vi "SQLite Get Calib.Parameters.vi"(8 "error in (no error)":errorcluster, 9 "VariableName":string, 10 "Order By":T1, 11 "Main":string="0") -> (0 "error out":errorcluster, 1 "Full Result":string[][](array[string]), 2 "Value":string, 3 "DBL Value":dbl, 4 "Results":string[](array[string]), 5 "Unit":string)   [LabVIEW 2017, in "SQLite.lvclass"]
doc: "get Calibration Parmeters.\n2015-11-05 10:00:32\n蒋松\njiangsong@outlook.com"
uses:
  SQLite.lvclass
  Order By.ctl
  SQLiteFileName.ctl
  TabelFullName.ctl
  <vilib>/Utility/error.llb/Trim Whitespace.vi
  <userlib>/LabSQL/LabSQL.lvlib
  <userlib>/sushu/sushu.lvlib
panel:
  in  "VI Ref":refnum<vi>
  in  "Alarm":bool=TRUE
  out "Boolean":bool
  in  "CMD":T2(ring)=enum."Read"
  out "Select SQL CMD":string
  # "Test-Force"
  # "ChannelItems"
  # "当是字符串格式的数字时，\n大于9后，排序会乱，\n1\n10\n2\n3\n...."
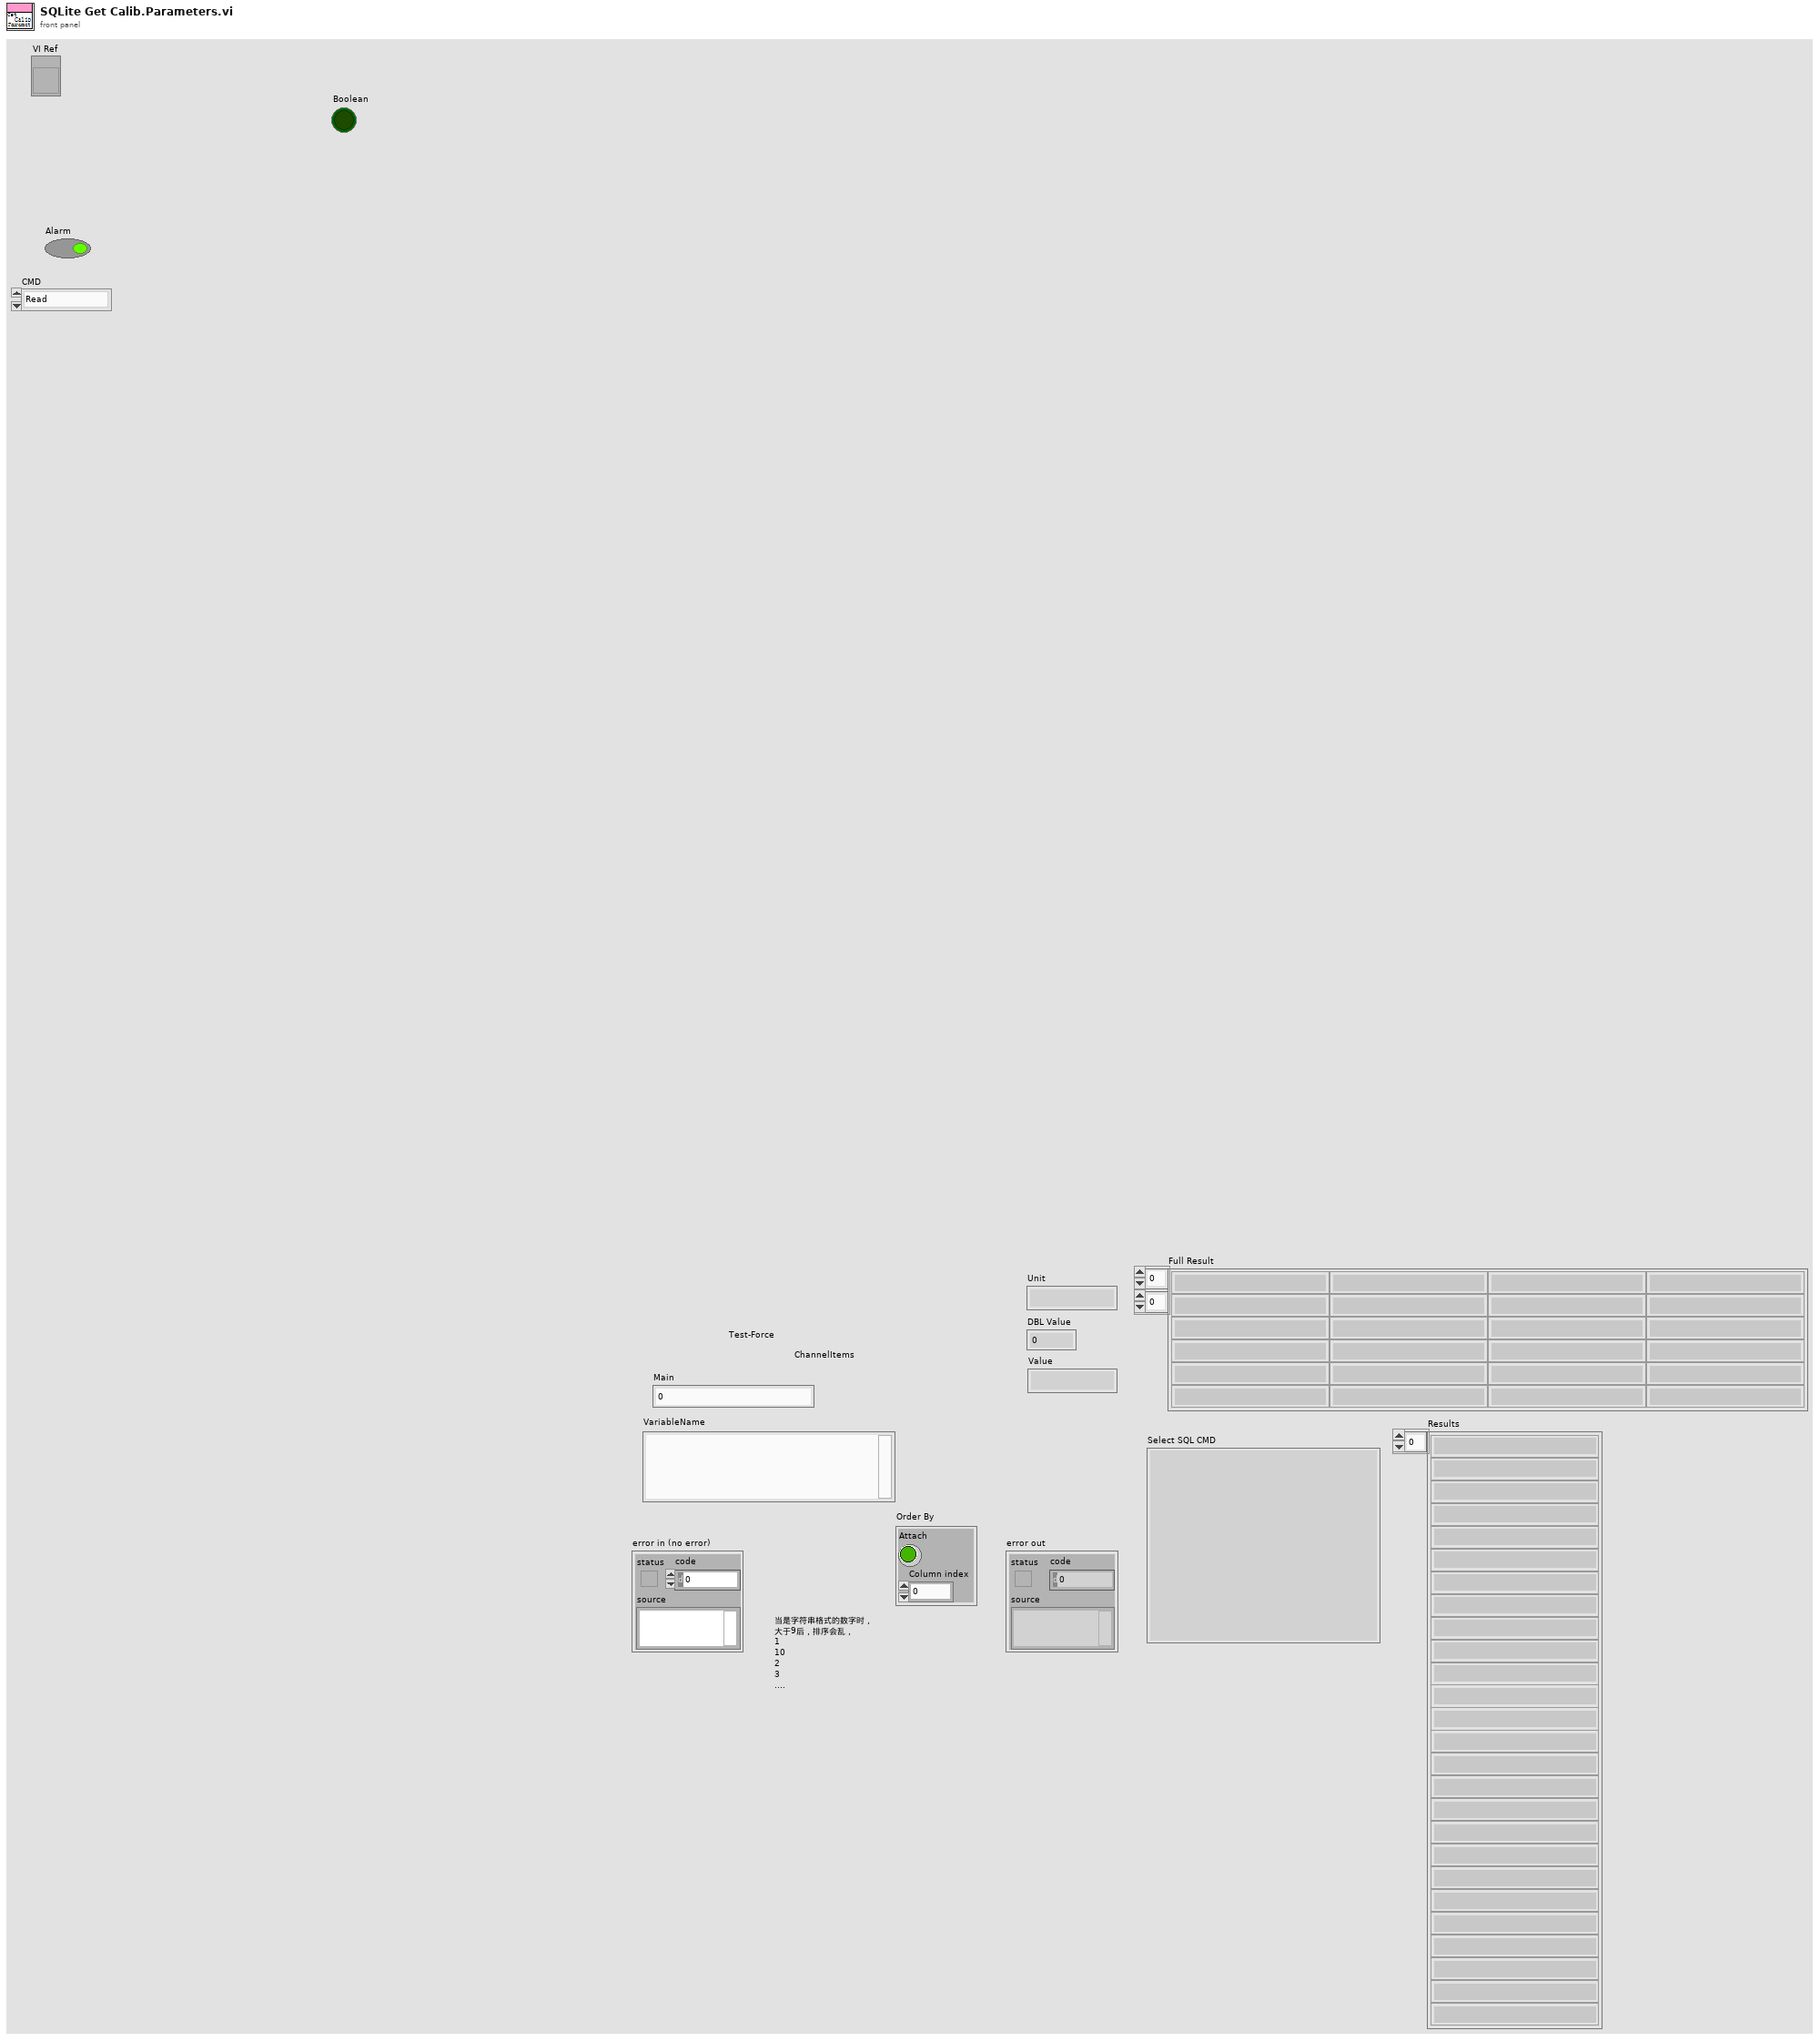
[diagram p1: front panel]
types:
  T1 = typedef "SQLite.lvclass/Order By.ctl" = cluster{"Attach":bool, "Column index":i32}
  T2 = enum16{"Initialize", "Read", "Write", "UnInitialize"}
  T3 = typedef "SQLite.lvclass/TabelFullName.ctl" = string
  T4 = typedef "SQLite.lvclass/SQLiteFileName.ctl" = string
  T5 = cluster{"Current VI Reference":refnum<vi>, "Close Panel on Exit?":bool}
  T6 = cluster{"Core":cluster{"Current VI Reference":refnum<vi>, "Close Panel on Exit?":bool}, "VI Name":string}
  T7 = enum16{"Other", "SQL2008", "SQLite", "Access", "MySQL"}
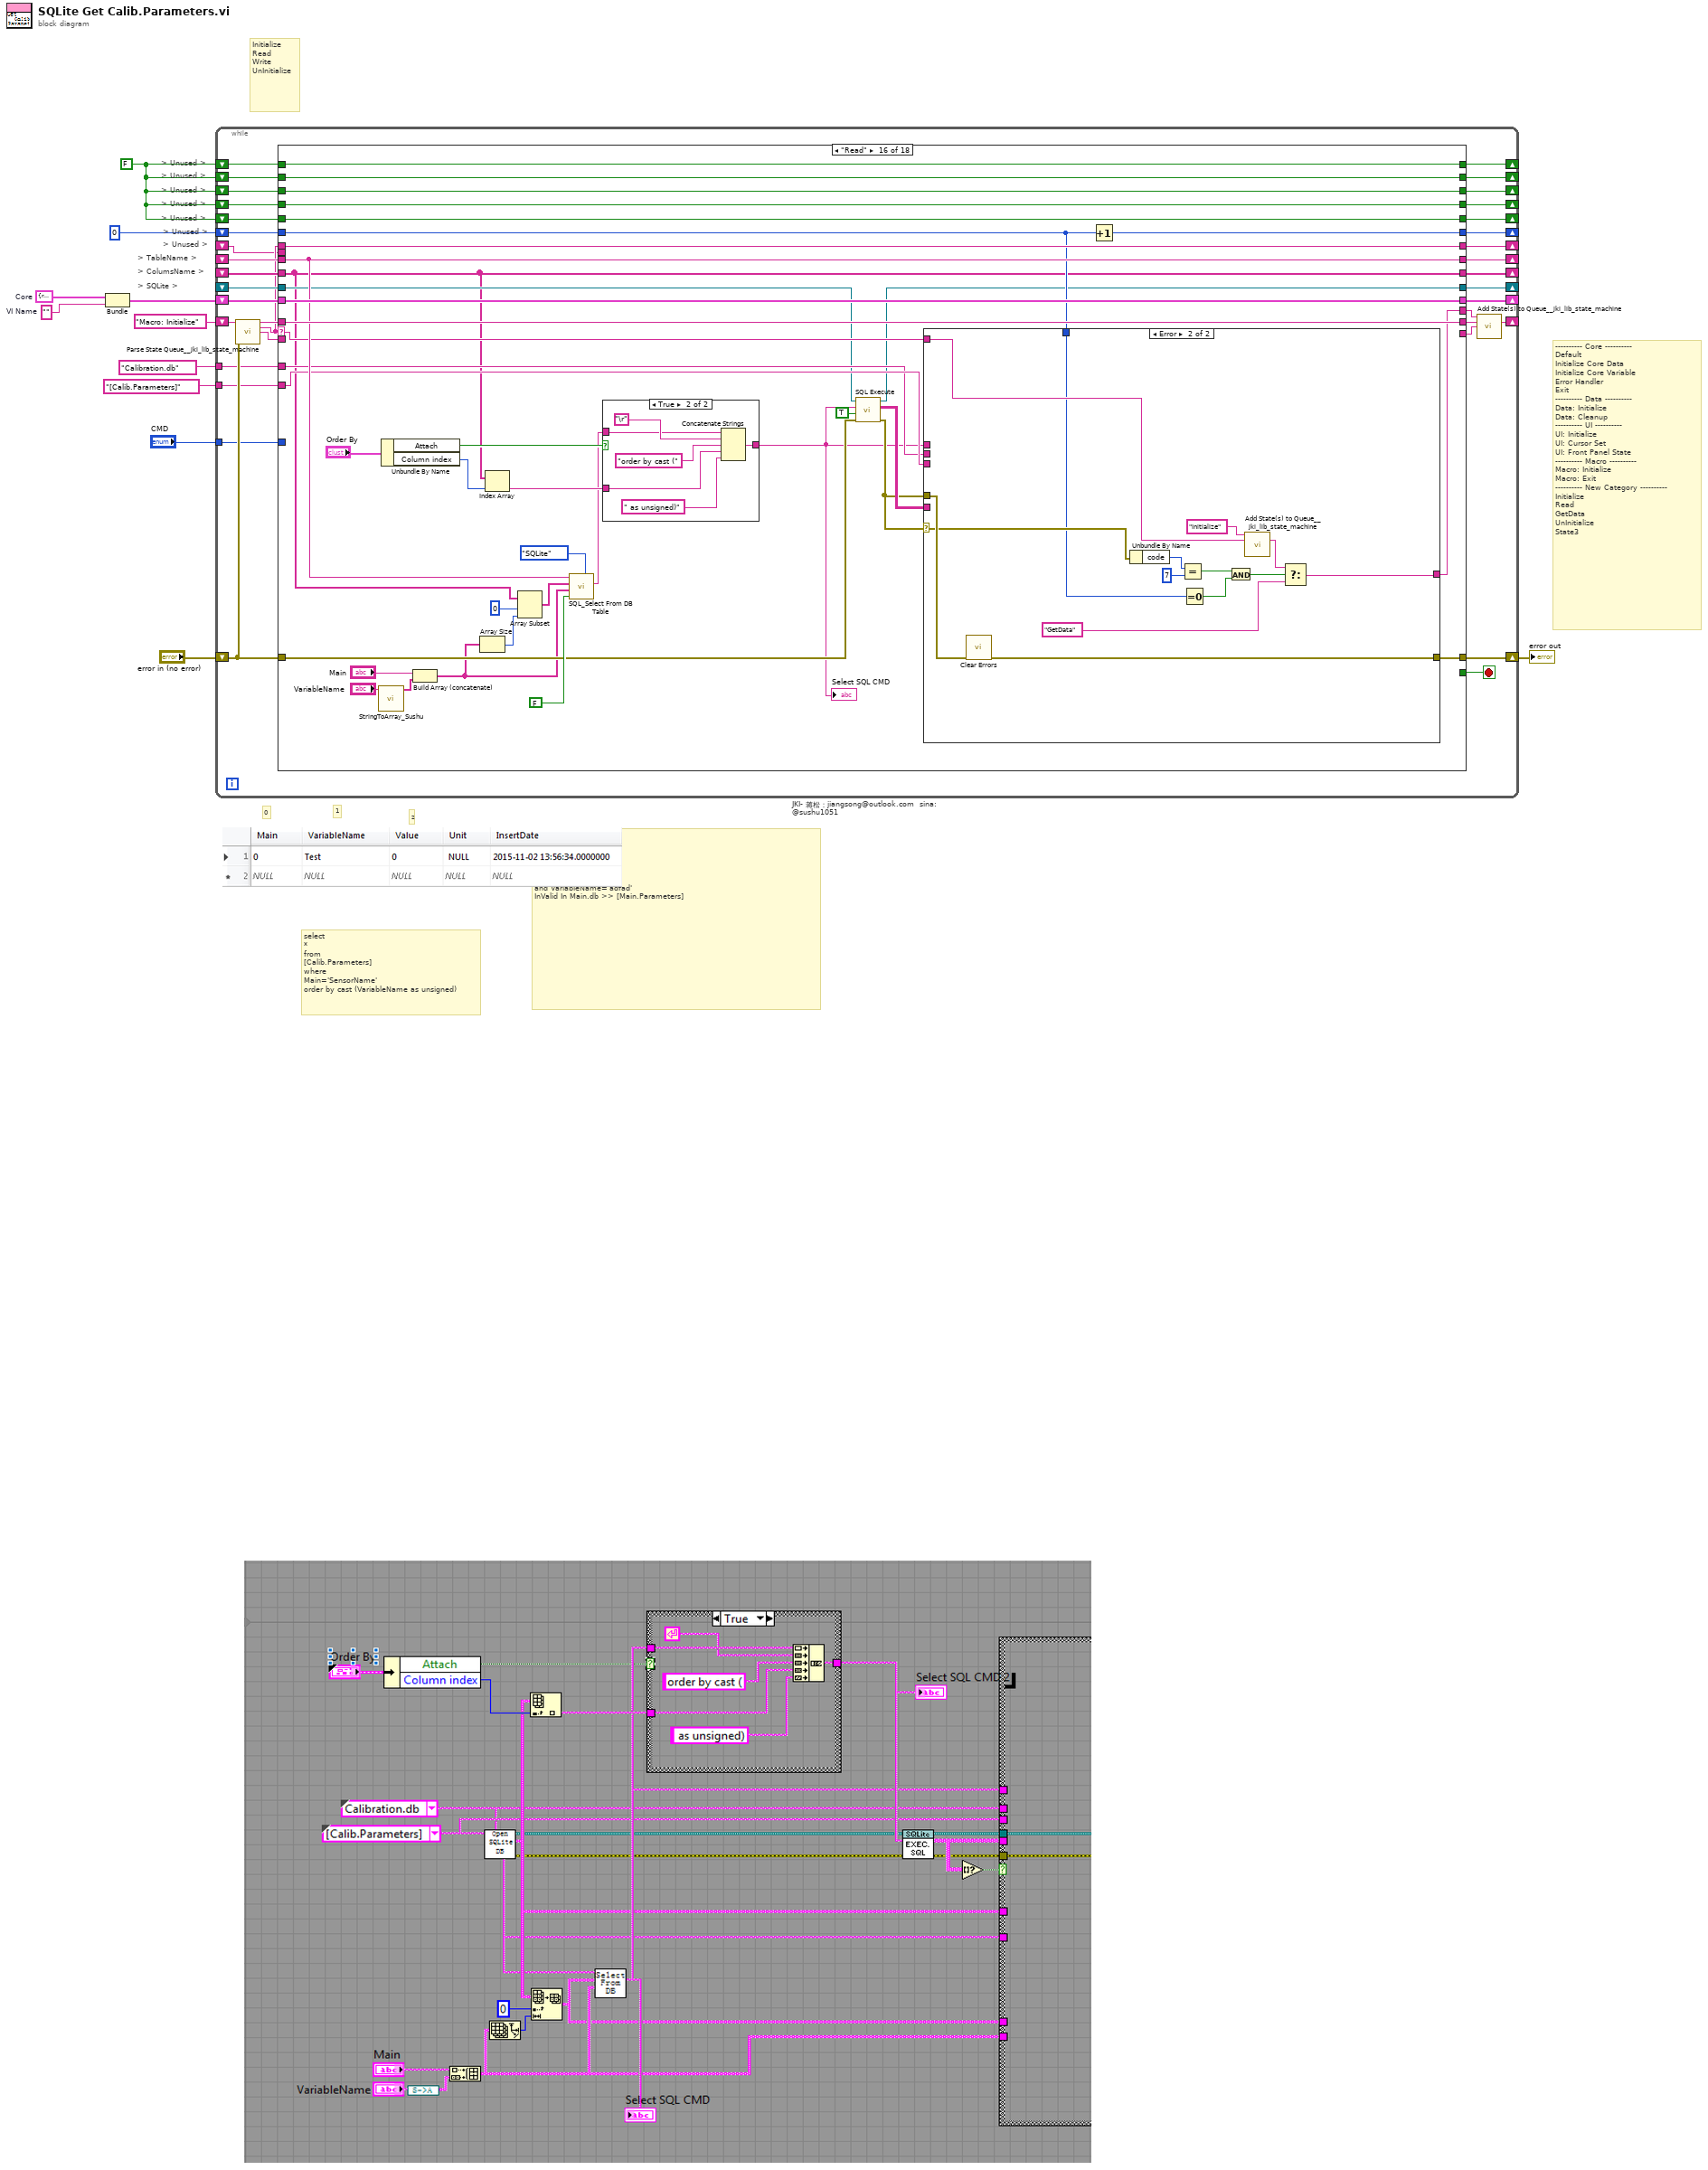
[diagram p0: block diagram]
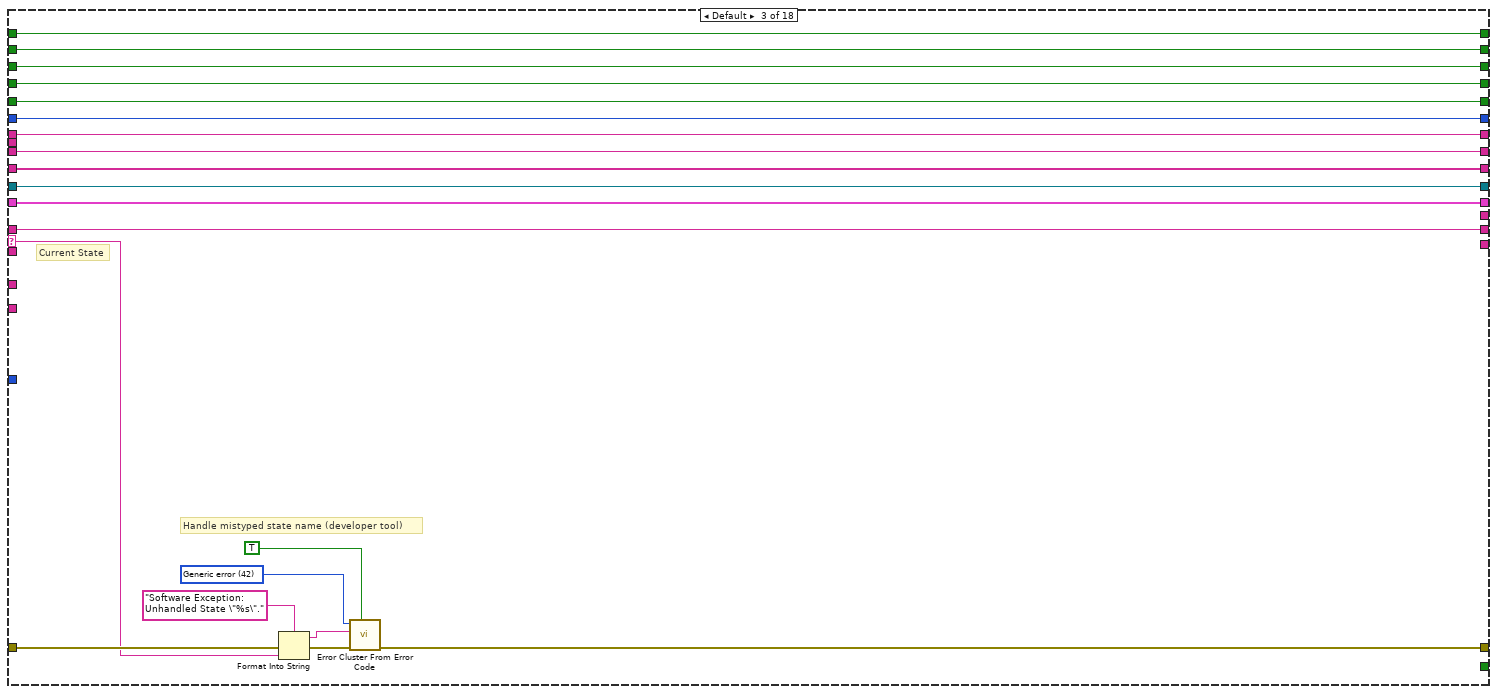
[diagram p4: hidden frame]
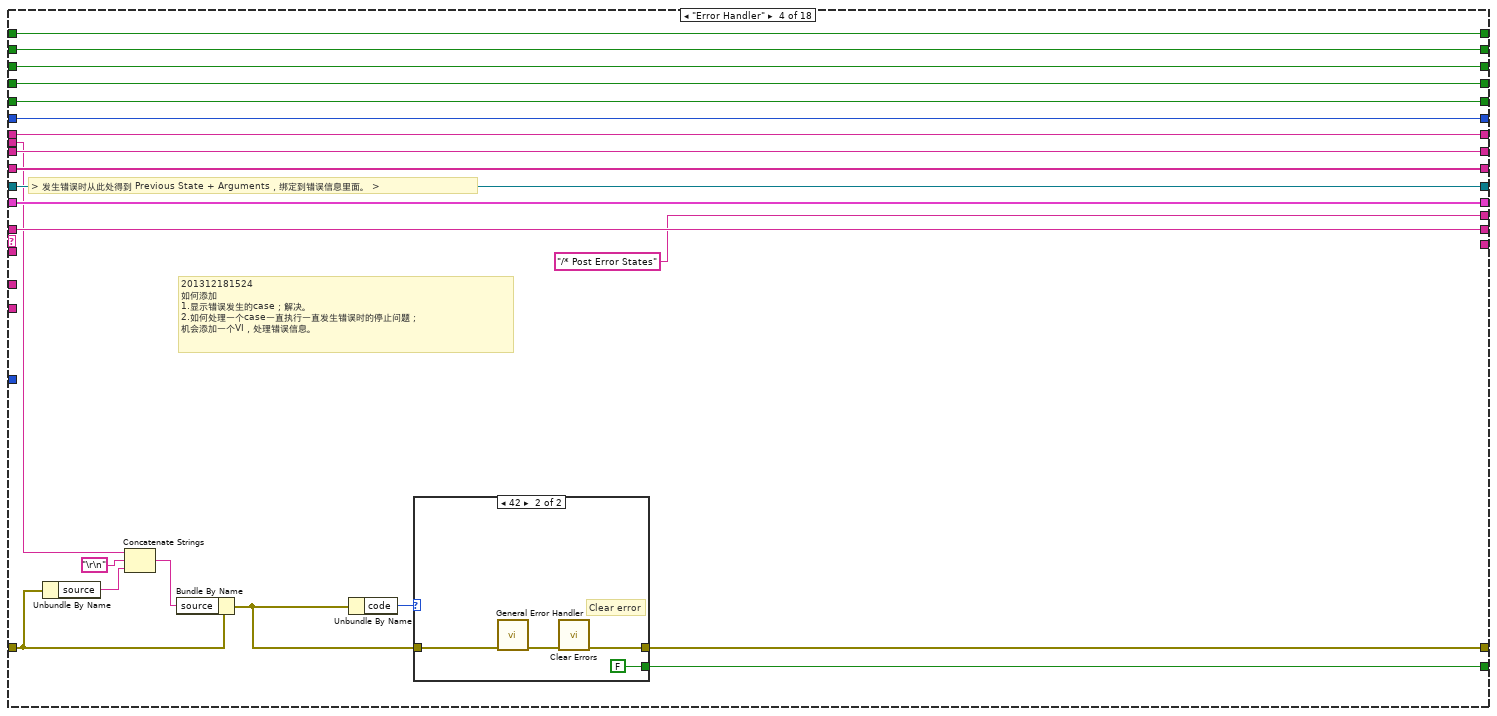
[diagram p5: hidden frame]
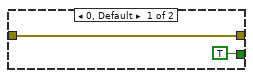
[diagram p6: hidden frame]
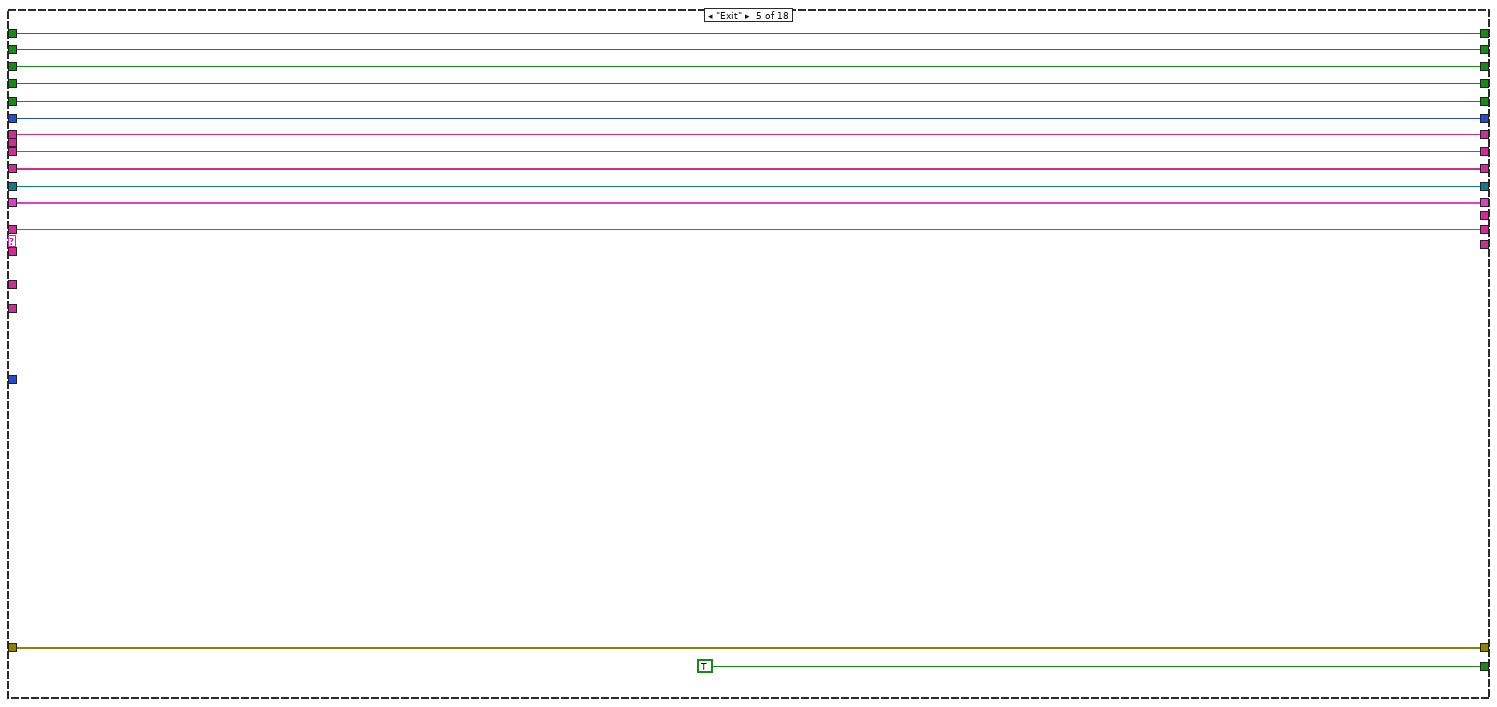
[diagram p7: hidden frame]
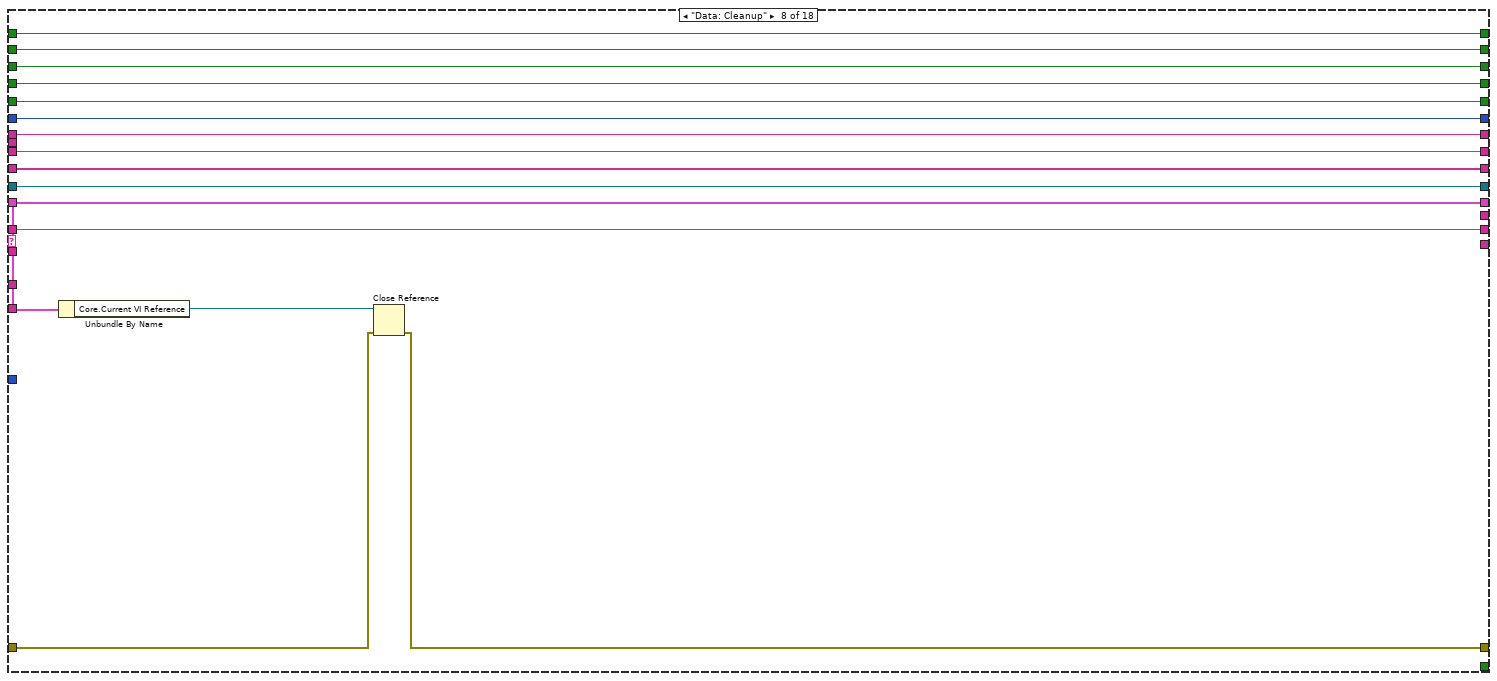
[diagram p10: hidden frame]
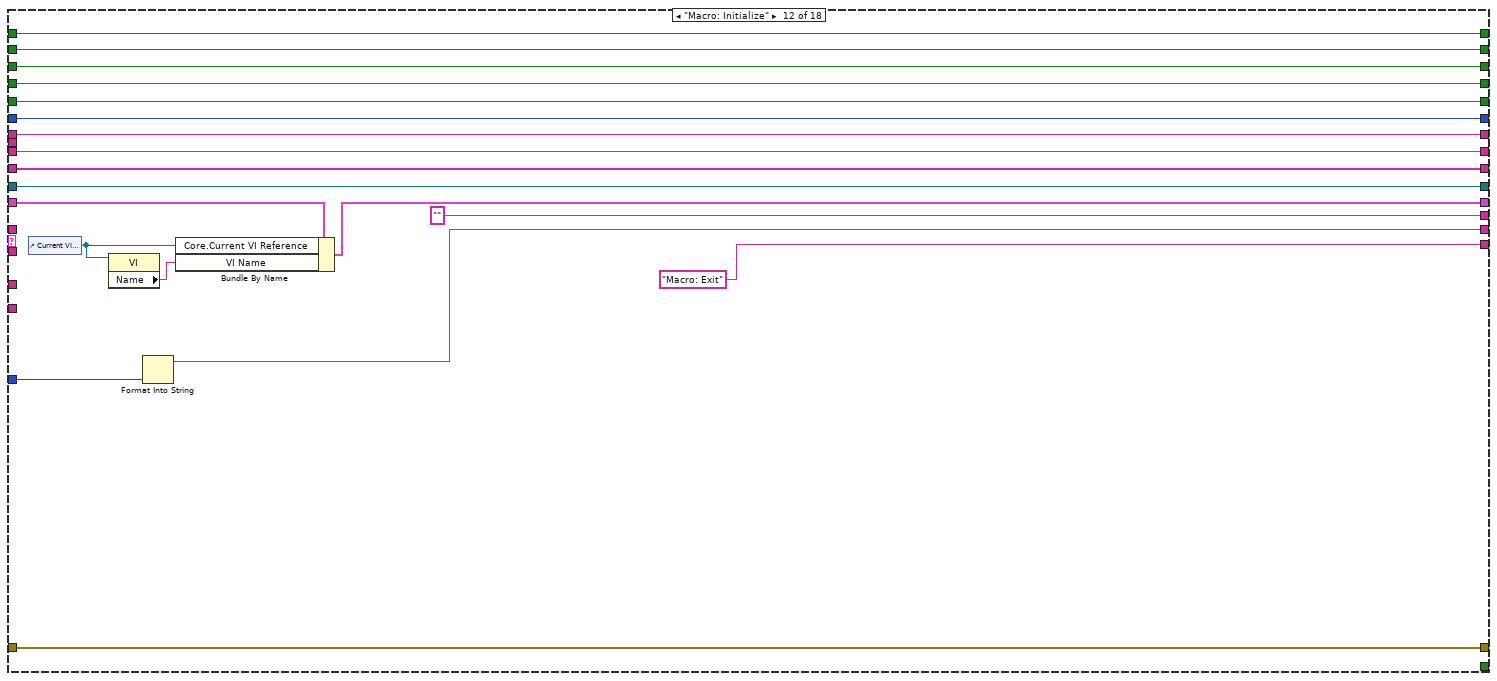
[diagram p14: hidden frame]
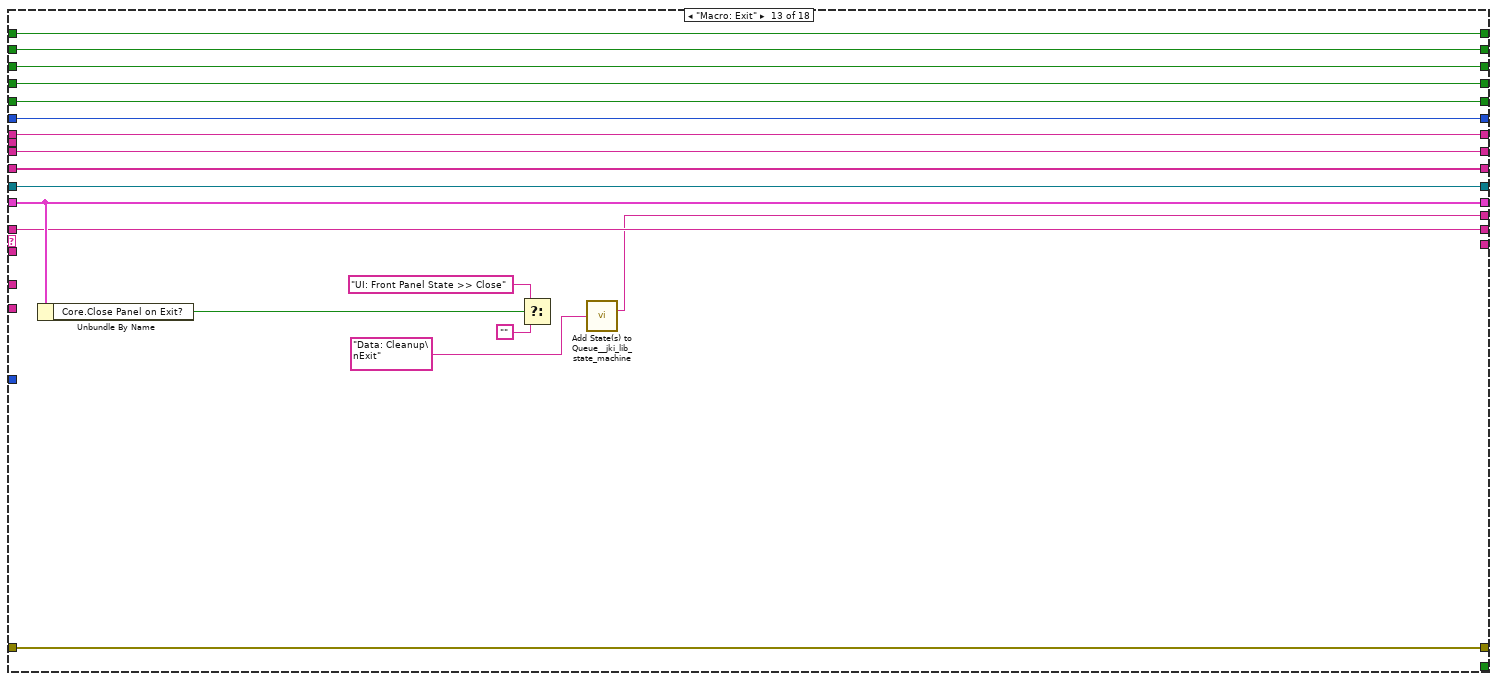
[diagram p15: hidden frame]
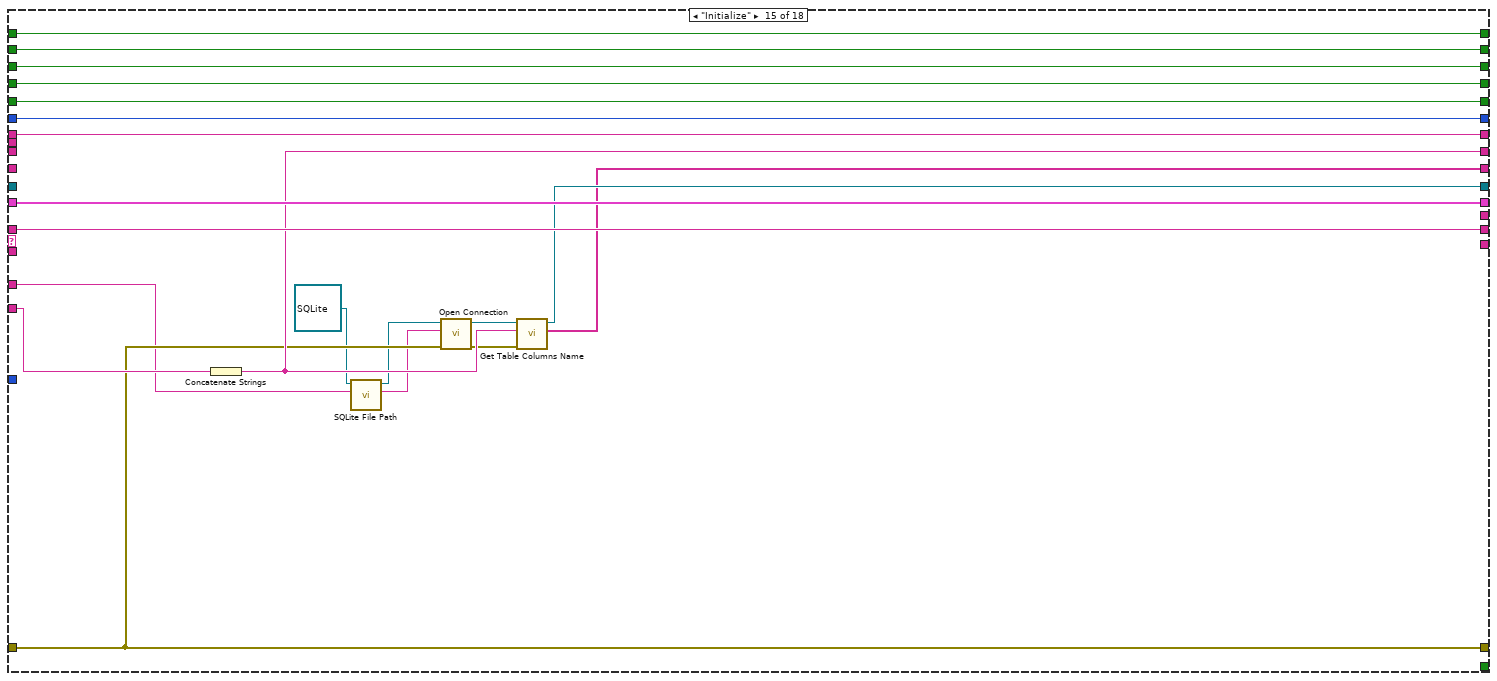
[diagram p17: hidden frame]
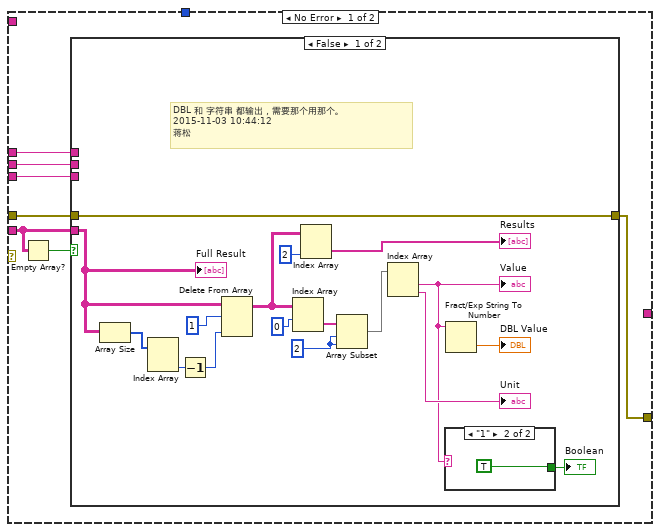
[diagram p19: hidden frame]
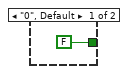
[diagram p20: hidden frame]
diagram:
  w11 = ""  # VI Name
  w10 = T5 {"Current VI Reference"=refnum, "Close Panel on Exit?"=FALSE}  # Core
  w6 = FALSE
  # "Initialize\nRead\nWrite\nUnInitialize"
  # "> Unused >"
  # "> Unused >"
  # "> Unused >"
  # "> Unused >"
  # "> Unused >"
  # "> Unused >"
  # "> SQLite >"
  # "> ColumsName >"
  # "> TableName >"
  # "> Unused >"
  # "---------- Core ----------\nDefault\nInitialize Core Data\nInitialize Core Variable\nError Handler\nExit\n---------- Data ----------\nData: Initialize\nData: Cleanup\n---------- UI ----------\nUI: Initialize\nUI: Cursor Set\nUI: Front Panel State\n---------- Macro ----------\nMacro: Initialize\nMacro: Exit\n---------- New Category ----------\nInitialize\nRead\nGetData\nUnInitialize\nState3"
  # "select\n*\nfrom\n[Calib.Parameters]\nwhere\nMain='SensorName'\norder by cast (VariableName as unsigned)"
  # "select\n*\nfrom\n[Main.Parameters]\nwhere\nMain='0'\nand VariableName='adfad'\nInValid In Main.db >> [Main.Parameters]"
  # "2"
  # "1"
  # "0"
  n1 = Bundle("Core"=w10, "VI Name"=w11) -> (w9:T6)  [unwired: 1 in]
  n2 = while "JKI- 蒋松：jiangsong@outlook.com  sina: @sushu1051" {
    shift-right: [w45] -> w1
    shift-left: "error in (no error)" -> [w43]
    shift-right: [w33] -> _
    shift-left: "Macro: Initialize" -> [w34]
    shift-right: [w40] -> _
    shift-left: _ -> [w42]
    shift-right: [w41] -> _
    shift-left: _ -> [w12]
    shift-right: [w35] -> _
    shift-left: w9 -> [w38]
    shift-right: [w36] -> _
    shift-left: _ -> [w29]
    shift-right: [w37] -> _
    shift-left: _ -> [w39]
    shift-right: [w28] -> _
    shift-left: 0 -> [w27]
    shift-right: [w20] -> _
    shift-left: w6 -> [w18]
    shift-right: [w19] -> _
    shift-left: w6 -> [w17]
    shift-right: [w23] -> _
    shift-left: w6 -> [w24]
    shift-right: [w22] -> _
    shift-left: w6 -> [w21]
    shift-right: [w25] -> _
    shift-left: w6 -> [w26]
    tunnel: "CMD" -> [w16]
    tunnel: T4 "Calibration.db" ("SQLiteFileName") -> [w15]
    tunnel: T3 "[Calib.Parameters]" ("TabelFullName") -> [w14]
    stop <- w44 stop-if-true
    n3 = call <vilib>:"Parse State Queue__jki_lib_state_machine.vi"("State Queue"=w34, "Error In (no error)"=w43) -> ("Remaining States"=w47:string, "Current State"=w13:string, "Arguments"=w46:string)  [unwired: 10 in, 1 out]
    n4 = case shown="\"Read\"" w13 {
      selector: w13 -> [_ _ w81 _ _ _ _ _ _ _ _ _ _ _ _ w306 _ _]
      tunnel: w47 -> [w60 w67 w80 w107 w128 w142 w156 w168 w183 w196 w209 _ w242 w259 w285 w323 w405 w420]
      tunnel: w46 -> [_ _ _ _ _ _ _ _ _ _ _ _ _ _ _ _ _ _]
      tunnel: [w59 w73 w82 w101 w130 w144 w158 w170 w185 w198 w211 w231 w249 w262 w270 w307 w393 w406] -> w45
      tunnel: w43 -> [w59 w73 w83 w111 w130 w144 w158 w171 w185 w198 w211 w231 w249 w262 w270 w300 w393 w407]
      tunnel: [w60 w67 w80 w107 w128 w142 w156 w168 w183 w196 w209 w217 w242 w259 w285 w323 w405 w420] -> w32
      tunnel: [_ _ _ w100 TRUE _ _ _ _ _ _ _ _ _ _ _ _ _] -> w44
      tunnel: w13 -> [w58 w72 w93 w115 w135 w148 w161 w176 w189 w202 w215 w234 w252 w265 w284 w308 w395 w419]
      tunnel: w42 -> [w57 w71 w92 w114 w134 w147 w160 w175 w188 w201 w214 w233 w251 w264 _ w312 w404 w418]
      tunnel: [w58 w72 w93 w115 w135 w148 w161 w176 w189 w202 w215 w234 w252 w265 w284 w308 w395 w419] -> w41
      tunnel: [w57 w71 w92 w114 w134 w147 w160 w175 w188 w201 w214 w233 w251 w264 w272 w312 w404 w418] -> w40
      tunnel: w39 -> [w56 w70 w91 w113 w133 w146 w159 w174 w187 w200 w213 w232 w250 w263 _ w291 w403 w417]
      tunnel: w29 -> [w54 w68 w90 w105 w129 w143 w157 w169 w184 w197 w210 w230 w243 w260 _ w303 w402 w409]
      tunnel: w38 -> [w55 w69 w89 w112 w132 w145 w149 w172 w186 w199 w212 w219 w244 w261 w283 w322 w401 w416]
      tunnel: [w56 w70 w91 w113 w133 w146 w159 w174 w187 w200 w213 w232 w250 w263 w273 w291 w403 w417] -> w37
      tunnel: [w54 w68 w90 w105 w129 w143 w157 w169 w184 w197 w210 w230 w243 w260 w274 w301 w402 w408] -> w36
      tunnel: [w55 w69 w89 w112 w132 w145 w149 w172 w186 w199 w212 w218 w244 w261 w283 w322 w401 w416] -> w35
      tunnel: [_ _ _ "/* Post Error States" _ _ _ _ _ _ _ "" w241 _ _ w305 _ _] -> w31
      tunnel: [_ _ _ _ _ _ _ _ _ _ _ "Macro: Exit" _ _ _ _ _ _] -> w30
      tunnel: w27 -> [w53 w66 w79 w104 w127 w141 w155 w167 w182 w195 w208 w229 w240 w258 w282 w304 w400 w415]
      tunnel: [w53 w66 w79 w104 w127 w141 w155 w167 w182 w195 w208 w229 w240 w258 w282 w317 w400 w415] -> w28
      tunnel: w17 -> [w51 w64 w77 w98 w125 w139 w153 w165 w180 w193 w206 w225 w238 w256 w277 w320 w399 w414]
      tunnel: w18 -> [w50 w63 w76 w97 w124 w138 w152 w164 w179 w192 w205 w224 w237 w255 w278 w319 w398 w413]
      tunnel: [w51 w64 w77 w98 w125 w139 w153 w165 w180 w193 w206 w225 w238 w256 w277 w320 w399 w414] -> w19
      tunnel: [w50 w63 w76 w97 w124 w138 w152 w164 w179 w192 w205 w224 w237 w255 w278 w319 w398 w413] -> w20
      tunnel: w21 -> [w49 w62 w75 w96 w123 w137 w151 w163 w178 w191 w204 w223 w236 w254 w279 w318 w397 w412]
      tunnel: w24 -> [w48 w61 w74 w95 w122 w136 w150 w162 w177 w190 w203 w222 w235 w253 w280 w309 w394 w411]
      tunnel: [w49 w62 w75 w96 w123 w137 w151 w163 w178 w191 w204 w223 w236 w254 w279 w318 w397 w412] -> w22
      tunnel: [w48 w61 w74 w95 w122 w136 w150 w162 w177 w190 w203 w222 w235 w253 w280 w309 w394 w411] -> w23
      tunnel: w26 -> [w52 w65 w78 w99 w126 w140 w154 w166 w181 w194 w207 w226 w239 w257 w281 w321 w396 w410]
      tunnel: [w52 w65 w78 w99 w126 w140 w154 w166 w181 w194 w207 w226 w239 w257 w281 w321 w396 w410] -> w25
      tunnel: w16 -> [_ _ _ _ _ _ _ _ _ _ _ w216 _ _ _ _ _ _]
      tunnel: w15 -> [_ _ _ _ _ _ _ _ _ _ _ _ _ _ w266 w310 _ _]
      tunnel: w14 -> [_ _ _ _ _ _ _ _ _ _ _ _ _ _ w275 w311 _ _]
      tunnel: w12 -> [_ _ _ w94 _ _ _ _ _ _ _ _ _ _ _ _ _ _]
      frame "Idle" {
      }
      frame "---------- Core ----------" {
      }
      frame Default {
        w85 = 42 items=["No error", "Argument error", "Memory is full", "Out of zone", "End of file", "File already open", "Generic file I/O error", "File not found", "File permission error", "Disk is full", "Duplicate path", "Too many files open", "System feature not enabled", "Resource file not found", "Cannot add resource", "Resource not found", "Image not found", "Image memory error", "Pen does not exist", "Config type invalid", "Config token not found", "Config parse error", "Config memory error", "Bad external code format", "Bad external code offset", "External code not present", "Null window", "Destroy window error", "Null menu", "Print aborted", "Bad print record", "Print driver error", "Windows error during printing", "Memory error during printing", "Print dialog error", "Generic print error", "Invalid device refnum", "Device not found", "Device parameter error", "Device unit error", "Cannot open device", "Device call aborted", "Generic error", "Cancelled by user", "Object ID too low", "Object ID too high", "Object not in heap", "Unknown heap", "Unknown object (invalid DefProc)", "Unknown object (DefProc not in table)", "Message out of range", "Invalid (null) method", "Unknown message", "Manager call not supported", "Bad address", "Network operation in progress", "Network operation timed out", "Connection is busy", "Network attribute not supported", "Network error", "Address in use", "System out of memory", "Connection aborted", "Connection refused", "Not connected", "Already connected", "Connection closed", "Initialization error (interapplication manager)", "Bad occurrence", "Wait on unbound occurrence handler", "Occurrence queue overflow", "Datalog type conflict", "Unused", "Unrecognized type (interapplication manager)", "Memory corrupt", "Failed to make temporary DLL", "Old CIN version", "Drag socket not found", "Failed to load drop-object", "Failed to register OLE object", "Failed to release OLE object", "Format specifier type mismatch", "Unknown format specifier", "Too few format specifiers", "Too many format specifiers", "Scan failed", "Newer CIN version", "Error converting to variant", "Runtime menu error", "Password tampered", "Variant attribute not found", "Incompatible variant data type", "Event data is not available", "Event Store is not present", "Occurrence is not found", "Event Queue is not created", "Event info is not available", "Refnum passed is NULL", "Error retrieving Class GUID", "Error retrieving CoClass GUID", "Error retrieving TypeLib GUID.", "Bad built application magic bytes.", "Specific driver is different from the specific driver associated with the Logical Name.", "There is no session opened to the class driver.", "Max Error", "MAX - Error with config objects", "MAX - Error loading configuration", "MAX - Group not supported"]
        # "Current State"
        # "Handle mistyped state name (developer tool)"
        n5 = Format Into String(format string="Software Exception: Unhandled State \"%s\"." ("message"), error in=w83, w81) -> (resulting string=w86:string, error out=w87:errorcluster)  [unwired: 1 in]
        n6 = call <vilib>:"Error Cluster From Error Code.vi"("show call chain? (False)"=TRUE, "error in (no error)"=w87, "error message (\"\")"=w86, "error code (0)"=w85) -> ("error out"=w82:errorcluster)  [unwired: 5 in]
      }
      frame "Error Handler" {
        # "> 发生错误时从此处得到 Previous State + Arguments，绑定到错误信息里面。 >"
        # "201312181524\n如何添加\n1.显示错误发生的case；解决。\n2.如何处理一个case一直执行一直发生错误时的停止问题；\n机会添加一个VI，处理错误信息。"
        # "Clear error"
        n7 = Unbundle By Name(w111) -> ("source"=w109:string)
        n8 = Concatenate Strings(w94, "\r\n", w109) -> (w108:string)
        n9 = Bundle By Name(cluster=w111, "source"=w108) -> (w102:errorcluster)
        n10 = Unbundle By Name(w102) -> ("code"=w103:i32)
        n11 = case shown="42" w103 {
          tunnel: [TRUE FALSE] -> w100
          tunnel: w102 -> [w117 w120]
          tunnel: [w117 w118] -> w101
          frame 0, Default {
          }
          frame 42 {
            n12 = call <vilib>:"General Error Handler.vi"("error in (no error)"=w120) -> ("error out"=w119:errorcluster)  [unwired: 10 in, 4 out]
            n13 = call <vilib>:"Clear Errors.vi"("error in (no error)"=w119) -> ("error out"=w118:errorcluster)  [unwired: 5 in, 1 out]
          }
        }
      }
      frame "Exit" {
      }
      frame "---------- Data ----------" {
      }
      frame "Data: Initialize" {
      }
      frame "Data: Cleanup" {
        n14 = Unbundle By Name(w172) -> ("Core.Current VI Reference"=w173:refnum<vi>)
        n15 = Close Reference(reference=w173, error in (no error)=w171) -> (error out=w170:errorcluster)
      }
      frame "---------- UI ----------" {
      }
      frame "UI: Initialize" {
      }
      frame "---------- Macro ----------" {
      }
      frame "Macro: Initialize" {
        n16 = control-ref of="Current VI Reference"() -> (w220:refnum<vi>)
        n17 = property class="VI"(reference=w220) -> ("Name"=w221:string)  [unwired: 1 in, 2 out]
        n18 = Format Into String(w216) -> (resulting string=w217:string)  [unwired: 3 in, 1 out]
        n19 = Bundle By Name(cluster=w219, "Core.Current VI Reference"=w220, "VI Name"=w221) -> (w218:T6)
      }
      frame "Macro: Exit" {
        n20 = Unbundle By Name(w244) -> ("Core.Close Panel on Exit?"=w245:bool)
        n21 = Select(t="UI: Front Panel State >> Close", s=w245, f="") -> ()  [unwired: 1 out]
        n22 = call <vilib>:"Add State(s) to Queue__jki_lib_state_machine.vi"("State(s) at Back (\"\")"="Data: Cleanup\nExit") -> ("States Out"=w241:string)  [unwired: 14 in]
      }
      frame "---------- New Category ----------" {
      }
      frame "Initialize" {
        n23 = Concatenate Strings(w275) -> (w272:string)
        n24 = call "SQLite File Path.vi"("SQLiteFileName"=w266, "SQLite in"=refnum<class "SQLite.lvclass"> refnum ("SQLite.lvclass")) -> ("string"=w269:string, "SQLite out"=w267:refnum<class "SQLite.lvclass">)  [unwired: 7 in, 1 out]
        n25 = call-dynamic "Open Connection.vi"("error in (no error)"=w270, "ConnectionString"=w269, "HostDB in"=w267) -> ("error out"=w271:errorcluster, "HostDB out"=w276:refnum<class "SQLite.lvclass">)  [unwired: 7 in]
        n26 = call-dynamic "Get Table Columns Name.vi"("error in (no error)"=w271, "TableName"=w272, "HostDB in"=w276) -> ("ColunmsList"=w273:string[], "HostDB out"=w274:refnum<class "SQLite.lvclass">)  [unwired: 4 in, 3 out]
      }
      frame "Read" {
        n27 = call <userlib>:"StringToArray_Sushu.vi"("State Queue"="VariableName") -> ("Array"=w298:string[])  [unwired: 8 in, 2 out]
        n28 = Unbundle By Name("Order By") -> ("Attach"=w293:bool, "Column index"=w292:i32)
        n29 = Build Array (concatenate)("Main", w298) -> (w295:string[])
        n30 = Array Size(array=w295) -> (size(s)=w314:i32)
        n31 = Index Array(array=w291, index=w292) -> (element=w294:string)
        n32 = Array Subset(array=w291, index=0, length=w314) -> (w316:string[])
        n33 = call <userlib>:"SQL_Select From DB Table.vi"("DB Type"=T7."SQLite", "Check ASCII?"=FALSE, "ColumnsValue"=w295, "ColumnsNameList"=w316, "TableName"=w312) -> ("Select SQL CMD"=w290:string)  [unwired: 6 in]
        n34 = case shown="True" w293 {
          tunnel: w290 -> [w324 w329]
          tunnel: w294 -> [_ w327]
          tunnel: [w324 w325] -> w289
          frame False {
          }
          frame True {
            n35 = Concatenate Strings(w329, "\r", "order by cast (" ("string"), w327, " as unsigned)" ("string")) -> (w325:string)
          }
        }
        "Select SQL CMD" <- w289
        n36 = call-dynamic "SQL Execute.vi"("error in (no error)"=w300, "Return Data (T)"=TRUE, "Command Text"=w289, "HostDB in"=w303) -> ("error out"=w299:errorcluster, "Table Control"=w302:string[][], "HostDB out"=w301:refnum<class "SQLite.lvclass">)  [unwired: 3 in, 2 out]
        n37 = case shown="Error" w299 {
          selector: w299 -> [_ w382]
          tunnel: w299 -> [w337 w392]
          tunnel: w289 -> [w335 _]
          tunnel: w302 -> [w334 _]
          tunnel: w311 -> [w333 _]
          tunnel: w310 -> [w332 _]
          tunnel: [w331 w391] -> w307
          tunnel: w306 -> [_ w381]
          tunnel: [_ w380] -> w305
          tunnel: w304 -> [_ w379]
          frame No Error {
            n38 = Empty Array?(array=w334) -> (empty?=w336:bool)
            n39 = case shown="False" w336 {
              tunnel: [w354 w362] -> w331
              tunnel: w337 -> [w354 w363]
              tunnel: w335 -> [_ w359]
              tunnel: w332 -> [_ w361]
              tunnel: w333 -> [_ w360]
              tunnel: w334 -> [w339 _]
              frame False {
                w346 = 2 ("index")
                # "DBL 和 字符串 都输出，需要那个用那个。\n2015-11-03 10:44:12\n蒋松"
                n40 = Array Size(array=w339) -> (size(s)=w340:i32[])
                n41 = Index Array(array=w340) -> (element #2=w341:i32)  [unwired: 2 in, 1 out]
                n42 = Decrement(x=w341) -> (x-1=w342:i32)
                n43 = Delete From Array(array=w339, length=1 ("disabled index (col)"), index (col)=w342) -> (array with subset deleted=w349:string[][])  [unwired: 1 in, 1 out]
                n44 = Index Array(array=w349, index (row)=0) -> (element=w344:string[])  [unwired: 1 in]
                n45 = Index Array(array=w349, index (col)=2 ("disabled index (col)")) -> (element=→"Results":string[])  [unwired: 1 in]
                n46 = Array Subset(array=w344, index=w346, length=w346) -> (w352:string[])
                n47 = Index Array(array=w352) -> (element #1=w338:string, element #2=→"Unit":string)  [unwired: 2 in]
                "Value" <- w338
                n48 = case shown="\"1\"" w338 {
                  tunnel: [FALSE ("Boolean") TRUE ("Boolean")] -> w353
                  frame "0", Default {
                  }
                  frame "1" {
                  }
                }
                "Boolean" <- w353
                n49 = Fract/Exp String To Number(string=w338) -> (number=→"DBL Value":dbl)  [unwired: 3 in, 1 out]
                "Full Result" <- w339
              }
              frame True {
                # "变量不存在，询问是否Insert。\n2015-11-03 09:57:10"
                n50 = case shown="True" "Alarm" {
                  tunnel: w363 -> [w364 w378]
                  tunnel: [w364 w377] -> w362
                  tunnel: w361 -> [_ w376]
                  tunnel: w360 -> [_ w375]
                  tunnel: w359 -> [_ w374]
                  tunnel: "VI Ref" -> [_ w365]
                  frame False {
                  }
                  frame True {
                    n51 = Concatenate Strings(w376) -> (w373:string)
                    n52 = Concatenate Strings(w375) -> (w372:string)
                    n53 = call <vilib>:"Build State String with Arguments__JKI_lib_State_Machine.vi"("Arguments (\"\")"=w372, "State"=w373) -> ("State with Arguments"=w370:string)  [unwired: 4 in]
                    n54 = Concatenate Strings(w374, "InValid In " ("Message"), w370) -> (w369:string)
                    n55 = call <userlib>:"Errors Handle Dialoge.vi"("VI Ref"=w365, "Cancel Text"="Ignore", "OK Text"="OK", "error in (no error)"=w378, "Title Text"="Select VariableName!", "Message"=w369) -> ("error out"=w377:errorcluster)  [unwired: 4 in, 1 out]
                  }
                }
              }
            }
          }
          frame Error {
            n56 = call <vilib>:"Clear Errors.vi"("error in (no error)"=w392) -> ("error out"=w391:errorcluster)  [unwired: 5 in, 1 out]
            n57 = Unbundle By Name(w382) -> ("code"=w389:i32)
            n58 = Equal?(x=w389, y=7) -> (x = y?=w387:bool)
            n59 = Equal To 0?(x=w379) -> (x = 0?=w386:bool)
            n60 = And(x=w387, y=w386) -> (x .and. y?=w385:bool)
            n61 = call <vilib>:"Add State(s) to Queue__jki_lib_state_machine.vi"("State(s) in Front (\"\")"="Initialize" ("Remaining States"), "State(s) in (\"\")"=w381) -> ("States Out"=w383:string)  [unwired: 13 in]
            n62 = Select(t=w383, s=w385, f="GetData") -> (s? t:f=w380:string)
          }
        }
        n63 = Increment(x=w304) -> (x+1=w317:i32)
      }
      frame "GetData" {
      }
      frame "UnInitialize" {
        n64 = call-dynamic "Close Connection.vi"("error in (no error)"=w407, "HostDB in"=w409) -> ("error out"=w406:errorcluster, "HostDB out"=w408:refnum<class "SQLite.lvclass">)  [unwired: 8 in]
      }
    }
    n65 = call <vilib>:"Add State(s) to Queue__jki_lib_state_machine.vi"("State(s) in Front (\"\")"=w31, "State(s) in (\"\")"=w32, "State(s) at Back (\"\")"=w30) -> ("States Out"=w33:string)  [unwired: 12 in]
  }
  "error out" <- w1
